vi "overlay transparency v2.vi"() -> ()   [LabVIEW 2015]
panel:
  out "Overlay plus background":T1(plugin-control)
  out "Overlay":T1(plugin-control)
  in  "Background image":path
  in  "image overlay":path
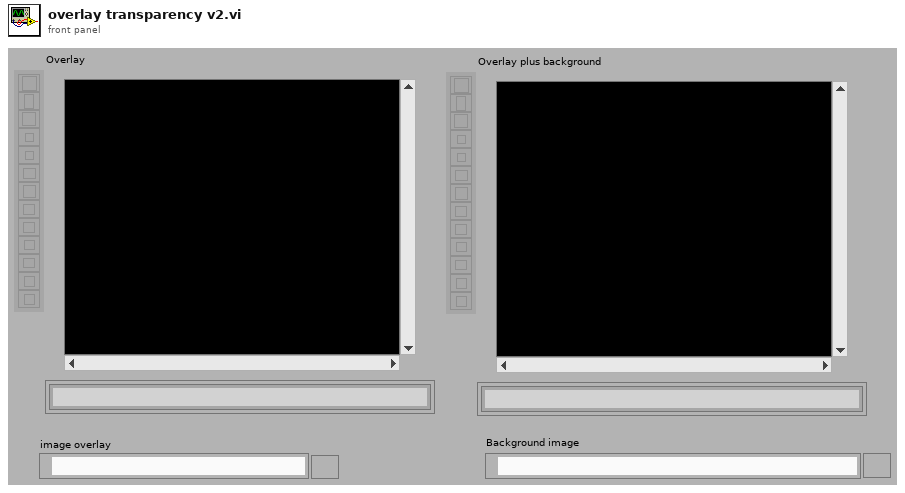
[diagram p1: front panel]
types:
  T1 = typedef "IMAQ Image.ctl" = refnum<image>
  T2 = typedef "Image Type" = u32
  T3 = typedef "imagedata.ctl" = cluster{"image type":i32, "image depth":i32, "image":u8[], "mask":u8[], "colors":u32[], "Rectangle":cluster{"left":i16, "top":i16, "right":i16, "bottom":i16}}
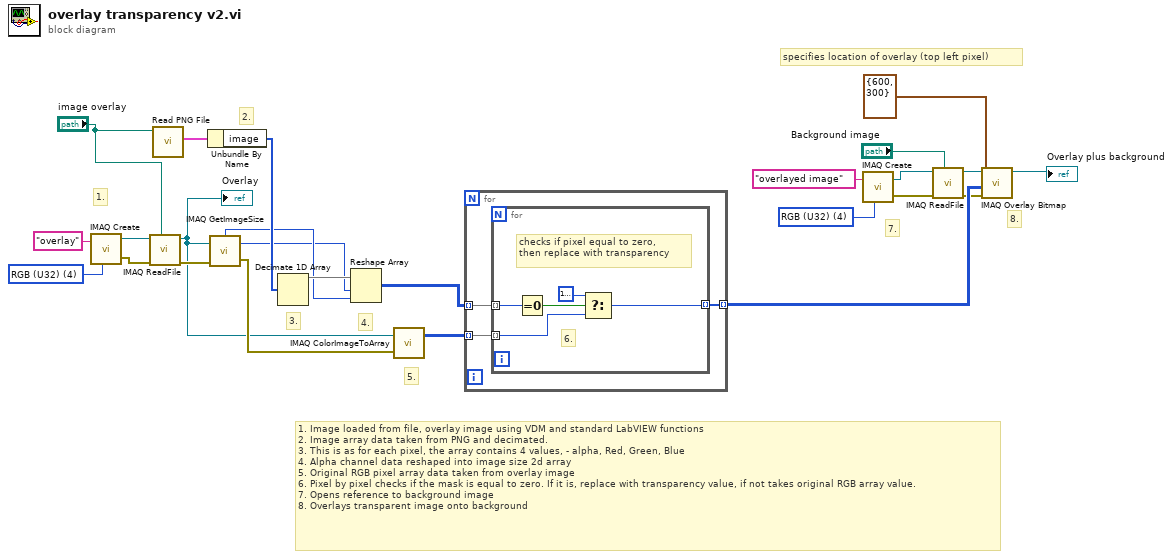
[diagram p0: block diagram]
diagram:
  w13 = T2 4 items=["Grayscale (U8)", "Grayscale (I16)", "Grayscale (SGL)", "Complex (CSG)", "RGB (U32)", "HSL (U32)", "RGB (U64)", "Grayscale (U16)"] ("Image Type")
  w15 = T2 4 items=["Grayscale (U8)", "Grayscale (I16)", "Grayscale (SGL)", "Complex (CSG)", "RGB (U32)", "HSL (U32)", "RGB (U64)", "Grayscale (U16)"] ("Image Type")
  # "specifies location of overlay (top left pixel)"
  # "8."
  # "7."
  # "1. Image loaded from file, overlay image using VDM and standard LabVIEW functions\n2. Image array data taken from PNG and decimated. \n3. This is as for each pixel, the array contains 4 values, - alpha, Red, Green, Blue\n4. Alpha channel data reshaped into image size 2d array\n5. Original RGB pixel array data taken from overlay image\n6. Pixel by pixel checks if the mask is equal to zero. If it is, replace with transparency value, if not takes original RGB array value.\n7. Opens reference to background image\n8. Overlays transparent image onto background"
  # "5."
  # "4."
  # "3."
  # "2."
  # "1."
  n1 = call "IMAQ Create"("Image Name"="overlay", "Image Type"=w15) -> ("New Image"=w21:T1, "error out"=w20:errorcluster)  [unwired: 3 in]
  n2 = call "IMAQ ReadFile"("File Path"="image overlay", "error in (no error)"=w20, "Image"=w21) -> ("error out"=w22:errorcluster, "Image Out"=w4:T1)  [unwired: 4 in, 3 out]
  "Overlay" <- w4
  n3 = call <vilib>:"Read PNG File.vi"("path to PNG file"="image overlay") -> ("image data"=w25:T3)  [unwired: 8 in, 2 out]
  n4 = Unbundle By Name(w25) -> ("image"=w24:u8[])
  n5 = call "IMAQ GetImageSize"("Image"=w4, "error in (no error)"=w22) -> ("Y Resolution"=w17:i32, "X Resolution"=w18:i32, "error out"=w6:errorcluster)  [unwired: 2 in]
  n6 = Decimate 1D Array(w24) -> (w23:u8[])  [unwired: 3 out]
  n7 = Reshape Array(w23, w17, w18) -> (w5:u8[][])
  n8 = call "IMAQ ColorImageToArray"("Image"=w4, "error in (no error)"=w6) -> ("Image Pixels (U32)"=w7:u32[][])  [unwired: 2 in, 2 out]
  n9 = for {
    tunnel: [w28] -> w8 mode=indexing
    tunnel: w5 -> [w27] mode=indexing
    tunnel: w7 -> [w26] mode=indexing
    n10 = for {
      tunnel: [w32] -> w28 mode=indexing
      tunnel: w27 -> [w31] mode=indexing
      tunnel: w26 -> [w30] mode=indexing
      # "6."
      # "checks if pixel equal to zero,\nthen replace with transparency"
      n11 = Equal To 0?(x=w31) -> (x = 0?=w33:bool)
      n12 = Select(t=u32 16777216, s=w33, f=w30) -> (s? t:f=w32:u32)
    }
  }
  n13 = call "IMAQ Create"("Image Name"="overlayed image", "Image Type"=w13) -> ("New Image"=w10:T1, "error out"=w14:errorcluster)  [unwired: 3 in]
  n14 = call "IMAQ ReadFile"("File Path"="Background image", "error in (no error)"=w14, "Image"=w10) -> ("error out"=w2:errorcluster, "Image Out"=w11:T1)  [unwired: 4 in, 3 out]
  n15 = call "IMAQ Overlay Bitmap"("error in (no error)"=w2, "Bitmap"=w8, "Top Left Point"=cluster{"X":i32, "Y":i32} {"X"=600, "Y"=300}, "Image"=w11) -> ("Image Out"=→"Overlay plus background":T1)  [unwired: 6 in, 1 out]
